vi "Get Status Section Reference.vi"(8 "error in":errorcluster, 11 "Ballard ARINC 429 ref":T1=18446744073709551615 format="%.0x") -> (0 "error out":errorcluster, 2 "status section reference":T1 format="%.0x", 3 "Ballard ARINC 429 ref out":T1 format="%.0x")   [LabVIEW 2020, in "Ballard ARINC 429 Scripting.lvlib"]
uses:
  <vilib>/NI VeriStand/Custom Device API/Custom Device Item Ref.ctl
  Constants.vi
  <vilib>/NI VeriStand/Custom Device Tools/Custom Device Utility Library/NI VeriStand - Search for Item by GUID.vi
  Ballard ARINC 429 Scripting.lvlib
  <vilib>/NI VeriStand/Custom Device Tools/Custom Device Utility Library/Custom Device Utility Library.lvlib
  <vilib>/NI VeriStand/Custom Device API/Custom Device API.lvlib
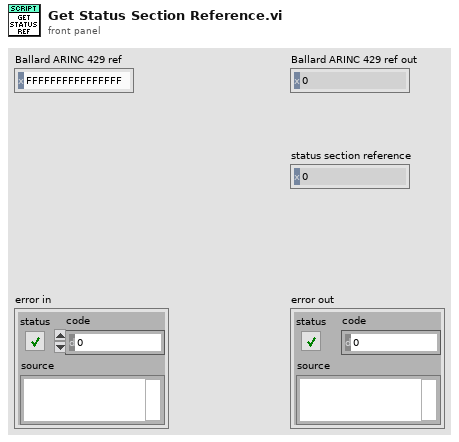
[diagram p1: front panel]
types:
  T1 = typedef "Custom Device API.lvlib/Custom Device Item Ref.ctl" = u64
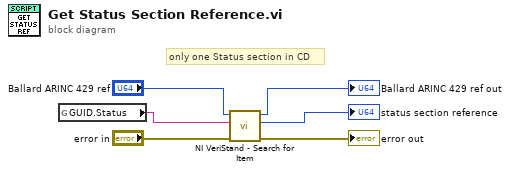
[diagram p0: block diagram]
diagram:
  # "only one Status section in CD"
  n1 = global read "Constants.vi" "GUID.Status"() -> (w4:string)
  n2 = call-poly <vilib>:"NI VeriStand - Search for Item.vi"("error in"="error in", "Item GUID"=w4, "Section Ref in"="Ballard ARINC 429 ref") -> ("error out"=→"error out":errorcluster, "Item Ref"=→"status section reference":T1, "Section Ref out"=→"Ballard ARINC 429 ref out":T1)  [unwired: 5 in, 1 out]
